vi "system type.vi"(8 "command":dbl=13.0 format="%.2f", 10 "system type":enum16{"1st ORDER", "2nd ORDER"}(ring), 11 "delta t (msec)":dbl=0.04 format="%.2f") -> (1 "response":dbl format="%.2f")   [LabVIEW 2016]
doc: "This subVI mimics an external system in software. You can choose between a first or second order system to which the PID sends its output for the Simple PID Demo.vi"
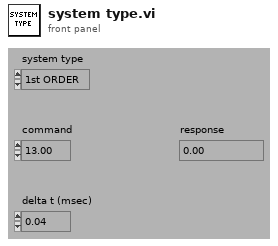
[diagram p1: front panel]
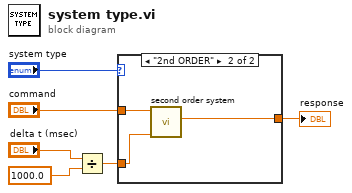
[diagram p0: block diagram]
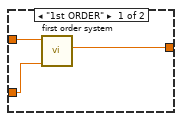
[diagram p2: hidden frame]
diagram:
  n1 = Divide(x="delta t (msec)", y=1000.0) -> (x/y=w3:dbl)
  n2 = case shown="\"2nd ORDER\"" "system type" {
    tunnel: "command" -> [w9 w12]
    tunnel: [w7 w11] -> w4
    tunnel: w3 -> [w8 w10]
    frame "1st ORDER" {
      n3 = call "first order system.vi"("delta t"=w8, "command"=w9) -> ("response"=w7:dbl)  [unwired: 9 in]
    }
    frame "2nd ORDER" {
      n4 = call "second order system.vi"("delta t"=w10, "command"=w12) -> ("response"=w11:dbl)  [unwired: 9 in]
    }
  }
  "response" <- w4
